vi "Init Dialog.vi"(6 "Allow to close? (T)":bool=TRUE, 7 "Dialog in":refnum<class "Dialog.lvclass">, 8 "error in (no error)":errorcluster, 9 "Timeout (-1)":i32=-1, 10 "Message":string, 11 "Dialog Title":string) -> (0 "error out":errorcluster, 3 "Dialog out":refnum<class "Dialog.lvclass">)   [LabVIEW 2012, in "Dialog.lvlib" / "Dialog.lvclass"]
doc: "This is an initialization VI to instantiate an object of Dialog class. (basic 1 button)."
uses:
  Dialog.lvclass
  Dialog.lvclass/Dialog.ctl
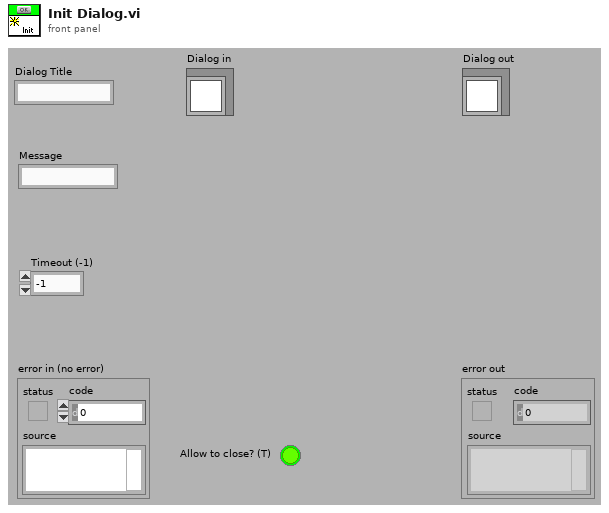
[diagram p1: front panel]
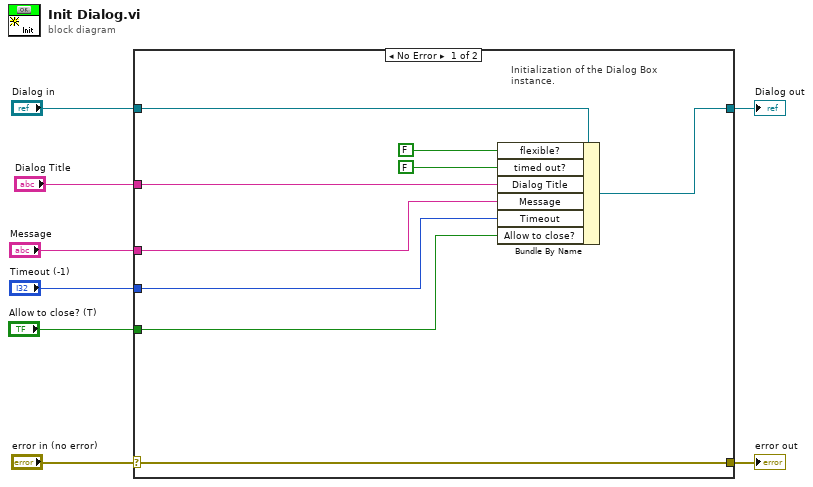
[diagram p0: block diagram]
diagram:
  n1 = case shown="No Error" "error in (no error)" {
    selector: "error in (no error)" -> [w9 w19]
    tunnel: [w9 w19] -> w7
    tunnel: [w16 w18] -> w5
    tunnel: "Dialog in" -> [w17 w18]
    tunnel: "Dialog Title" -> [w15 _]
    tunnel: "Message" -> [w14 _]
    tunnel: "Timeout (-1)" -> [w12 _]
    tunnel: "Allow to close? (T)" -> [w11 _]
    frame No Error {
      # "Initialization of the Dialog Box\ninstance."
      n2 = Bundle By Name(cluster=w17, "flexible?"=FALSE, "timed out?"=FALSE, "Dialog Title"=w15, "Message"=w14, "Timeout"=w12, "Allow to close?"=w11) -> (w16:refnum<class "Dialog.lvclass">)
    }
    frame Error {
    }
  }
  "error out" <- w7
  "Dialog out" <- w5
